vi "Create Array of n-Exp Fit Constraints.vi"(8 "Error In":errorcluster, 9 "parameter bounds in":T1, 10 "Offset Resolution":dbl, 11 "Guess Parameters in":dbl[](array[numeric])) -> (0 "Error Out":errorcluster, 1 "Array of parameter bounds":T2(array[cluster]), 3 "Guess Offset Array":dbl[](array[numeric]))   [LabVIEW 2021, in "Fits.lvlib"]
uses:
  Fits.lvlib
  Arrays/Linear Ramp End Options.ctl
  Arrays/Arrays.lvlib
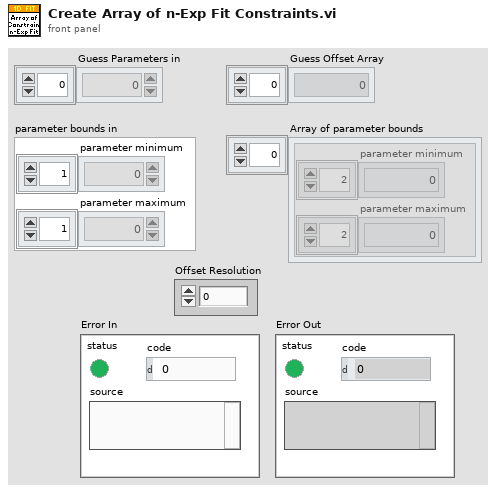
[diagram p1: front panel]
types:
  T1 = cluster{"parameter minimum":dbl[], "parameter maximum":dbl[]}
  T2 = cluster{"parameter minimum":dbl[], "parameter maximum":dbl[]}[]
  T3 = typedef "Arrays.lvlib/Linear Ramp End Options.ctl" = enum16{"Include Min/Exclude Max", "Exclude Min/Include Max", "Include Both Ends", "Exclude Both Ends"}
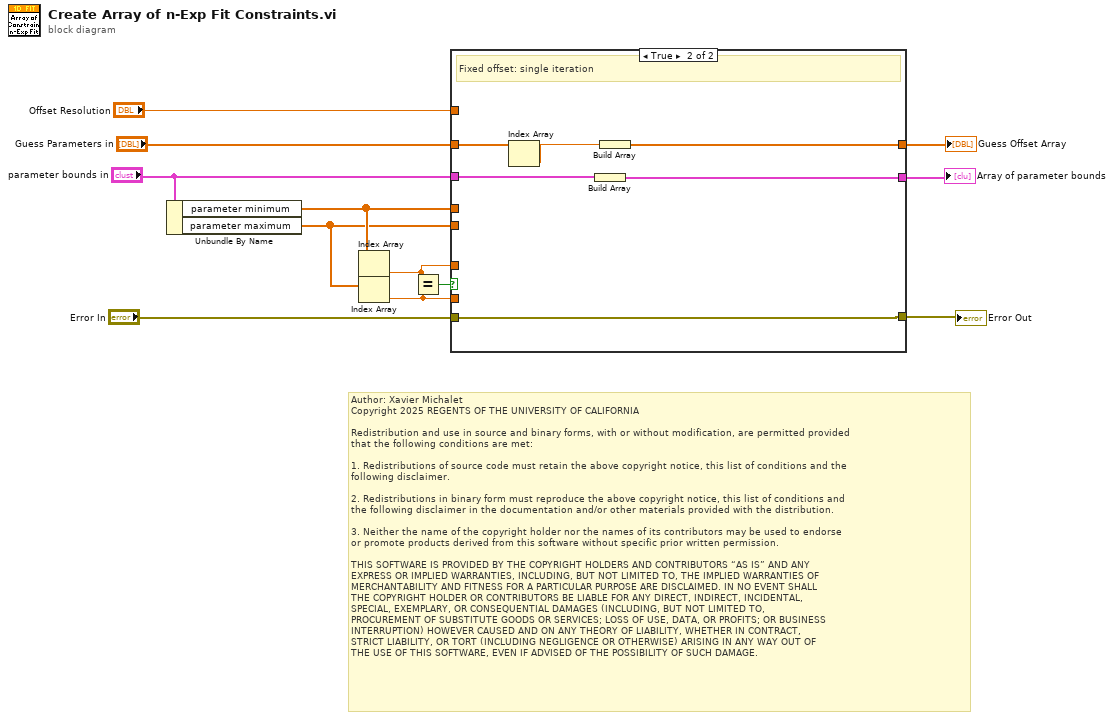
[diagram p0: block diagram]
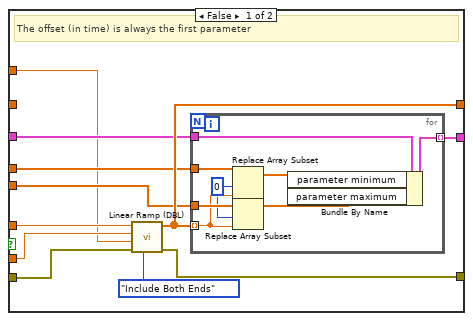
[diagram p2: hidden frame]
diagram:
  # "Author: Xavier Michalet\nCopyright 2025 REGENTS OF THE UNIVERSITY OF CALIFORNIA\n\nRedistribution and use in source and binary forms, with or without modification, are permitted provided\nthat the following conditions are met:\n\n1. Redistributions of source code must retain the above copyright notice, this list of conditions and the\nfollowing disclaimer.\n\n2. Redistributions in binary form must reproduce the above copyright notice, this list of conditions and\nthe following disclaimer in the documentation and/or other materials provided with the distribution.\n\n3. Neither the name of the copyright holder nor the names of its contributors may be used to endorse \nor promote products derived from this software without specific prior written permission.\n\nTHIS SOFTWARE IS PROVIDED BY THE COPYRIGHT HOLDERS AND CONTRIBUTORS “AS IS” AND ANY \nEXPRESS OR IMPLIED WARRANTIES, INCLUDING, BUT NOT LIMITED TO, THE IMPLIED WARRANTIES OF\nMERCHANTABILITY AND FITNESS FOR A PARTICULAR PURPOSE ARE DISCLAIMED. IN NO EVENT SHALL\nTHE COPYRIGHT HOLDER OR CONTRIBUTORS BE LIABLE FOR ANY DIRECT, INDIRECT, INCIDENTAL, \nSPECIAL, EXEMPLARY, OR CONSEQUENTIAL DAMAGES (INCLUDING, BUT NOT LIMITED TO, \nPROCUREMENT OF SUBSTITUTE GOODS OR SERVICES; LOSS OF USE, DATA, OR PROFITS; OR BUSINESS\nINTERRUPTION) HOWEVER CAUSED AND ON ANY THEORY OF LIABILITY, WHETHER IN CONTRACT, \nSTRICT LIABILITY, OR TORT (INCLUDING NEGLIGENCE OR OTHERWISE) ARISING IN ANY WAY OUT OF\nTHE USE OF THIS SOFTWARE, EVEN IF ADVISED OF THE POSSIBILITY OF SUCH DAMAGE."
  n1 = Unbundle By Name("parameter bounds in") -> ("parameter minimum"=w4:dbl[], "parameter maximum"=w3:dbl[])
  n2 = Index Array(array=w4) -> (element=w6:dbl)  [unwired: 1 in]
  n3 = Index Array(array=w3) -> (element=w5:dbl)  [unwired: 1 in]
  n4 = Equal?(x=w6, y=w5) -> (x = y?=w12:bool)
  n5 = case shown="True" w12 {
    tunnel: "Guess Parameters in" -> [_ w37]
    tunnel: [w20 w35] -> w10
    tunnel: "parameter bounds in" -> [w19 w33]
    tunnel: [w16 w34] -> w8
    tunnel: "Offset Resolution" -> [w15 _]
    tunnel: w6 -> [w21 _]
    tunnel: w5 -> [w22 _]
    tunnel: w4 -> [w18 _]
    tunnel: w3 -> [w17 _]
    tunnel: "Error In" -> [w14 w32]
    tunnel: [w13 w32] -> w1
    frame False {
      # "The offset (in time) is always the first parameter"
      n6 = call "Linear Ramp (DBL).vi"("Options"=Linear_Ramp_End_Options."Include Both Ends", "Error In"=w14, "Delta"=w15, "Max"=w22, "Min"=w21) -> ("Error Out"=w13:errorcluster, "Ramp"=w20:dbl[])  [unwired: 4 in, 1 out]
      n7 = for {
        tunnel: w20 -> [w29] mode=indexing
        tunnel: w19 -> [w27]
        tunnel: w18 -> [w31]
        tunnel: w17 -> [w30]
        tunnel: [w24] -> w16 mode=indexing
        w28 = 0 ("index")
        n8 = Replace Array Subset(array=w31, new element=w29, index=w28) -> (w26:dbl[])
        n9 = Replace Array Subset(array=w30, new element=w29, index=w28) -> (w25:dbl[])
        n10 = Bundle By Name(cluster=w27, "parameter minimum"=w26, "parameter maximum"=w25) -> (w24:T1)
      }
    }
    frame True {
      # "Fixed offset: single iteration"
      n11 = Index Array(array=w37) -> (element=w36:dbl)  [unwired: 1 in]
      n12 = Build Array(w33) -> (w34:T2)
      n13 = Build Array(w36) -> (w35:dbl[])
    }
  }
  "Guess Offset Array" <- w10
  "Array of parameter bounds" <- w8
  "Error Out" <- w1
